vi "Validate Variable Header.vi"(8 "error in (no error)":errorcluster, 11 "PUBLISH in":refnum<class "PUBLISH.lvclass">) -> (0 "error out":errorcluster, 1 "valid?":bool, 3 "PUBLISH out":refnum<class "PUBLISH.lvclass">)   [LabVIEW 2013, in "MQTT_Control_Packets.lvlib" / "PUBLISH.lvclass"]
uses:
  PUBLISH.lvclass
  PUBLISH.lvclass/PUBLISH.ctl
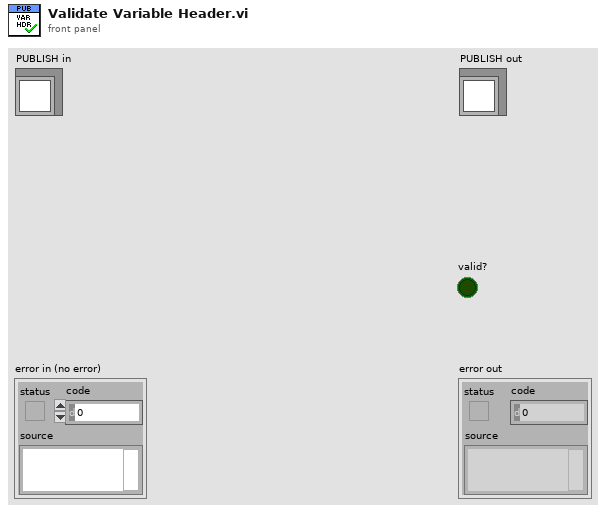
[diagram p1: front panel]
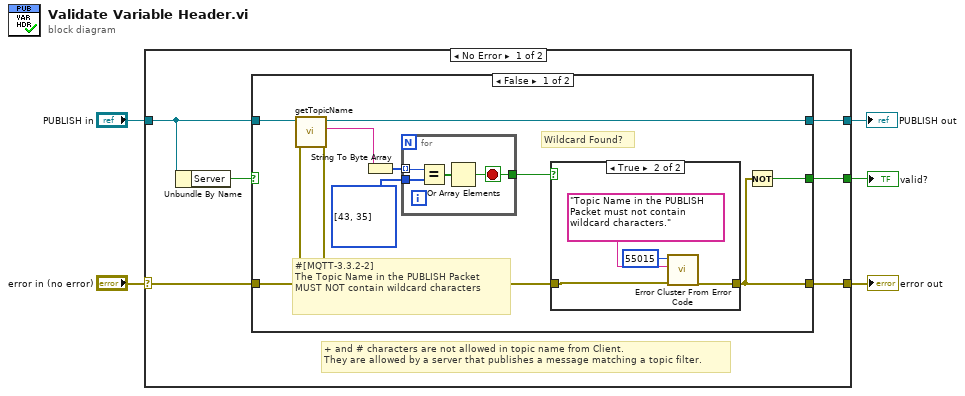
[diagram p0: block diagram]
diagram:
  n1 = case shown="No Error" "error in (no error)" {
    selector: "error in (no error)" -> [w10 w34]
    tunnel: "PUBLISH in" -> [w7 w35]
    tunnel: [w11 w35] -> w3
    tunnel: [w8 w34] -> w2
    tunnel: [w9 _] -> w1
    frame No Error {
      # "+ and # characters are not allowed in topic name from Client.\nThey are allowed by a server that publishes a message matching a topic filter."
      n2 = Unbundle By Name(w7) -> ("Server"=w6:bool)
      n3 = case shown="False" w6 {
        selector: w6 -> [_ w31]
        tunnel: [w21 w33] -> w11
        tunnel: w10 -> [w20 w32]
        tunnel: [w16 w31] -> w9
        tunnel: [w13 w32] -> w8
        tunnel: w7 -> [w12 w33]
        frame False {
          # "Wildcard Found?"
          # "#[MQTT-3.3.2-2]\nThe Topic Name in the PUBLISH Packet MUST NOT contain wildcard characters"
          n4 = call "getTopicName.vi"("error in (no error)"=w20, "PUBLISH in"=w12) -> ("error out"=w14:errorcluster, "Topic"=w19:string, "PUBLISH out"=w21:refnum<class "PUBLISH.lvclass">)  [unwired: 7 in]
          n5 = String To Byte Array(string=w19) -> (unsigned byte array=w18:u8[])
          n6 = for {
            tunnel: w18 -> [w30] mode=indexing
            tunnel: u8[] [43, 35] ("unsigned byte array") -> [w29]
            tunnel: [w27] -> w15
            stop <- w27 stop-if-true
            n7 = Equal?(x=w30, y=w29) -> (x = y?=w28:bool[])
            n8 = Or Array Elements(Boolean array=w28) -> (logical OR=w27:bool)
          }
          n9 = case shown="True" w15 {
            tunnel: w14 -> [w22 w25]
            tunnel: [w22 w26] -> w13
            frame False {
            }
            frame True {
              n10 = call <vilib>:"Error Cluster From Error Code.vi"("error in (no error)"=w25, "error message (\"\")"="Topic Name in the PUBLISH Packet must not contain wildcard characters.", "error code (0)"=55015) -> ("error out"=w26:errorcluster)  [unwired: 6 in]
            }
          }
          n11 = Not(x=w13) -> (.not. x?=w16:bool)
        }
        frame True {
        }
      }
    }
    frame Error {
    }
  }
  "error out" <- w2
  "PUBLISH out" <- w3
  "valid?" <- w1
